vi "diceSimulator.vi"() -> ()   [LabVIEW 2018]
panel:
  in  "stop":bool
  in  "Roll":bool
  out "Numeric":dbl
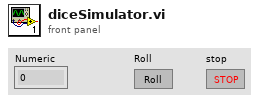
[diagram p1: front panel]
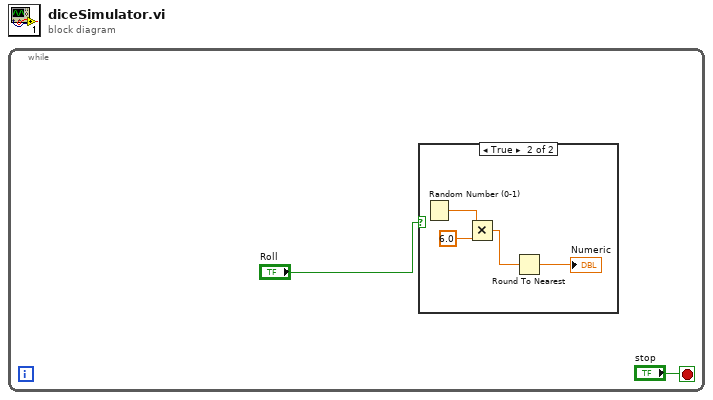
[diagram p0: block diagram]
diagram:
  n1 = while {
    stop <- "stop" stop-if-true
    n2 = case shown="True" "Roll" {
      frame False {
      }
      frame True {
        n3 = Random Number (0-1)() -> (number: 0 to 1=w6:dbl)
        n4 = Multiply(x=w6, y=6.0) -> (x*y=w4:dbl)
        n5 = Round To Nearest(number=w4) -> (nearest integer value=→"Numeric":dbl)
      }
    }
  }
